vi "Data Unsubscribed.vi"(8 "error in (no error)":errorcluster, 10 "Groups":string[](array[string]), 11 "LocalGraphBuffer in":refnum<class "LocalGraphBuffer.lvclass">) -> (0 "error out":errorcluster, 3 "LocalGraphBuffer out":refnum<class "LocalGraphBuffer.lvclass">)   [LabVIEW 2020, in "VolatusGUIElements.lvlib" / "LocalGraphBuffer.lvclass"]
uses:
  LocalGraphBuffer.lvclass
  LocalGraphBuffer.lvclass/LocalGraphBuffer.ctl
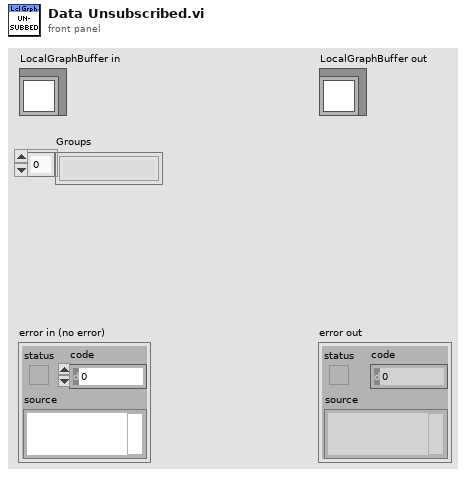
[diagram p1: front panel]
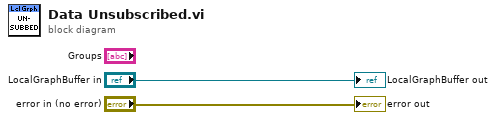
[diagram p0: block diagram]
diagram:
  "error out" <- "error in (no error)"
  "LocalGraphBuffer out" <- "LocalGraphBuffer in"
